vi "ServoCommand.vi"(8 "value":bool, 9 "command":u8(ring)=1 items=["Hold"=1, "Servo"=2, "HLock"=3], 10 "HighSpeedEServer":refnum<k24>, 11 "error in (no error)":errorcluster) -> (3 "error out":errorcluster)   [LabVIEW 2013, in "UnderAutomation.Yaskawa.lvlib"]
uses:
  UnderAutomation.Yaskawa.lvlib
  C:/Users/fg/Documents/Yaskawa.vi/LabVIEW_2024/UnderAutomation.Yaskawa/lib/UnderAutomation.Yaskawa.dll
  LabVIEW_2024/UnderAutomation.Yaskawa/lib/UnderAutomation.Yaskawa.dll
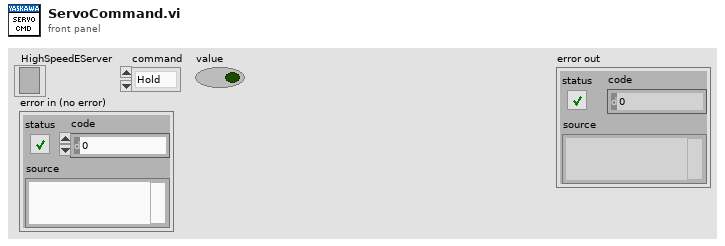
[diagram p1: front panel]
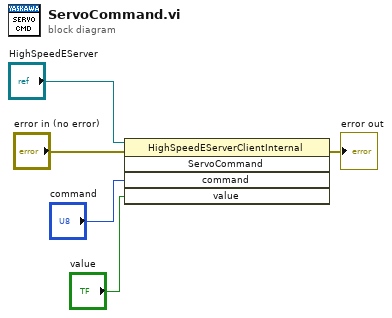
[diagram p0: block diagram]
diagram:
  n1 = invoke class="HighSpeedEServerClientInternal" method="ServoCommand"(reference="HighSpeedEServer", error in="error in (no error)", "command"="command", "value"="value") -> (error out=→"error out":errorcluster)  [unwired: 1 in, 4 out]
